vi "save results array.vi"(9 "save results":bool, 10 "test results in":T1, 11 "test results array":T1[](array[typedef])) -> (3 "test results array out":T1[](array[typedef]))   [LabVIEW 2020]
uses:
  controls/test results.ctl
  controls/step_type.ctl
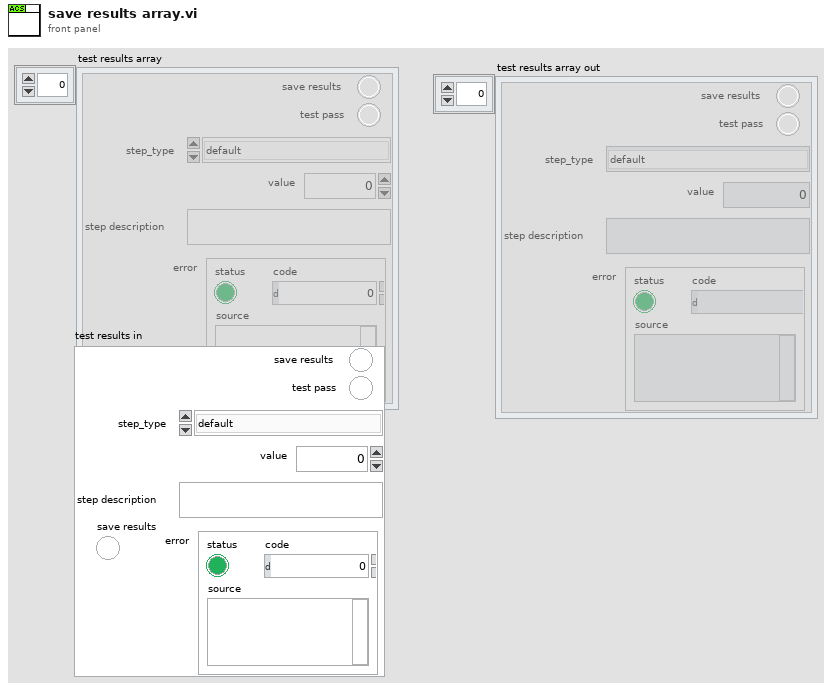
[diagram p1: front panel]
types:
  T1 = typedef "test results.ctl" = cluster{"test pass":bool, "step_type":T2, "value":dbl, "step description":string, "error":errorcluster, "save results":bool}
  T2 = typedef "step_type.ctl" = enum16{"default", "prompt", "sequence#", "12V_1_power supply on_off", "12V_2_power supply on_off", "set_hipot_V", "set_hipot_I_limit", "set_hipot_ramping (sec)", "set hipot_hold_time", "read_hipot_V", "read_hipot_I", "set_daq", "read_daq", "flash uds", "wait (sec)", "record_pass_fail", "ac_charge_test", "dc_400V_charging", "HAPS Heater Output", "HAPS Compressor Output", "stop_test", "error_exit"}
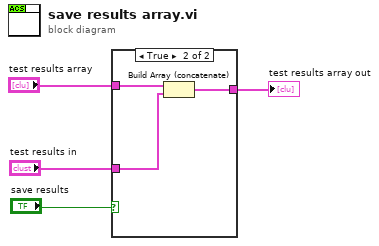
[diagram p0: block diagram]
diagram:
  n1 = case shown="True" "save results" {
    tunnel: "test results array" -> [w5 w8]
    tunnel: [w5 w7] -> w2
    tunnel: "test results in" -> [_ w6]
    frame False {
    }
    frame True {
      n2 = Build Array (concatenate)(w8, w6) -> (w7:T1[])
    }
  }
  "test results array out" <- w2
